vi "Stitching-Validate rows selection.vi"(7 "Loaded data":string[][](array[string]), 11 "Selected rows indexes in":i32[](array[numeric])) -> (3 "Selected rows indexes":i32[](array[numeric]))   [LabVIEW 2013]
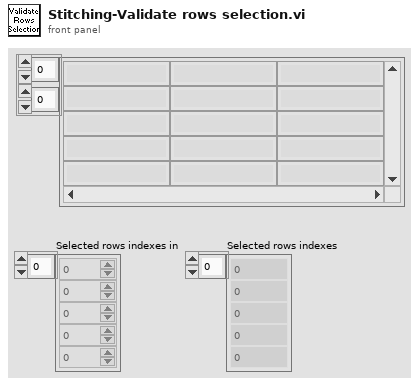
[diagram p1: front panel]
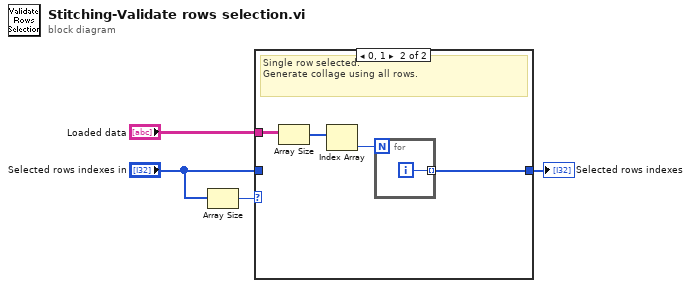
[diagram p0: block diagram]
diagram:
  n1 = Array Size(array="Selected rows indexes in") -> (size(s)=w4:i32)
  n2 = case shown="0, 1" w4 {
    tunnel: [w5 w6] -> w2
    tunnel: "Selected rows indexes in" -> [w5 _]
    tunnel: "Loaded data" -> [_ w9]
    frame Default {
      # "Multiple rows selected.\nGenerate collage using the specified rows only."
    }
    frame 0, 1 {
      # "Single row selected.\nGenerate collage using all rows."
      n3 = Array Size(array=w9) -> (size(s)=w8:i32[])
      n4 = Index Array(array=w8) -> (element=w7:i32)  [unwired: 1 in]
      n5 = for {
        N: w7 -> [_]
        tunnel: [w10] -> w6 mode=indexing
        i -> [w10]
      }
    }
  }
  "Selected rows indexes" <- w2
